vi "Getting Started with OAT (Offline, Analog Tacho) .vi"() -> ()   [LabVIEW 2017]
doc: "<B>DESCRIPTIONS</B>:\nThis VI demonstrates how to perform basic order analysis functions such as speed calculation, vibration level measurement, spectral map, order power spectrum, and order magnitude and phase. It uses simulated signals or loads previously recorded signals acquired with Log Data (Analog Tacho, DAQmx).vi for offline analysis. \n\n<B>INSTRUCTIONS</B>:\n1. Select tab page <B>Generate Signal</B> to use simulated signal or tab page <B>Load Data</B> to load logged signal.\n2. When using simulated signal, specify the <B>sampling info</B>, <B>signal rotating speed</B> and <B>order components</B> contained in the signal.\n3. When using recorded data, select the data file to load.\n4. Run the VI.\n5. On the <B>Time Waveform and Speed Profile</B> tab, select the signal of interest in <B>select channel</B> and specify the <B>Start</B> and <B>Duration</B> of the signal to calculate sound or vibration level. Run the VI again to make the changes take effect.\n6. On the <B>Colormap</B> tab, select the signal of interest in <B>select channel</B>. Use the <B>plot type</B> control to change the type of colormap. Specify the <B>time segment</B> and <B>spectra settings</B> to get a better view of the colormap. Run the VI again to make the changes take effect.\n7. On the <B>Order Power Spectrum</B> tab, specify the <B>Start</B> and <B>Duration</B> of the signal to calculate the order power spectrum. Specify the <B>window type</B>, <B>block size</B> and <B>averaging parameters</B> to improve the order power spectrum calculation and display. Run the VI again to make the changes take effect.\n<B>Note</B>: when the <B>Duration</B> of the signal is too short, there may not be an order power spectrum output. In this case, you should increase the duration or decrease the <B>block size</B> to get the order power spectrum results.\n8. On the <B>Magnitude and Phase</B> tab, select the signal of interest in <B>select channel</B> and specify the order to calculate magnitude and phase in <B>orders to compute</B>. Change the <B>magnitude view</B> and <B>view</B> to gain desired magnitude and phase display formats. Run the VI again to make the changes take effect.\n\n<B>ORDER ANALYSIS VIs USED IN THIS EXAMPLE</B>:\n1. SVL Scale Voltage to EU.vi\n2. OAT Analog Tacho Process.vi\n3. SVL RMS Level.vi\n4. SVL Peak Level.vi\n5. OAT Spectral Map.vi\n6. OAT Convert to Even Angle Signal.vi\n7. OAT Order Power Spectrum.vi\n8. OAT Order Magnitude and Phase.vi\n9. SVL Unit Conversion.vi"
uses:
  <vilib>/addons/_NISVFA/_Shared subVIs/Controls/svc_Channel Info.ctl
  <vilib>/addons/_NISVFA/_Shared subVIs/Controls/svc_Engineering Units Text Ring.ctl
  <vilib>/addons/_NISVFA/_Shared subVIs/Controls/svc_Weighting Filter Text Ring.ctl
  <vilib>/addons/_XControls/Colormap/SVX Colormap.xctl
  <vilib>/addons/_NISVFA/_Shared subVIs/Common/svc_Set SV Channel Info.vi
  <vilib>/addons/_NISVFA/_Shared subVIs/Common/svc_Set SV Channel Info (variant).vi
  <vilib>/addons/_NISVFA/_Shared subVIs/Common/SVL Set dB Reference (variant).vi
  <vilib>/addons/_NISVFA/_Shared subVIs/Common/svc_Caller VI Returned in Error Source.vi
  <vilib>/addons/_NISVFA/_Shared subVIs/Common/svc_Engineering Units to Unit Label.vi
  <vilib>/addons/_NISVFA/_Shared subVIs/Common/svc_Set dB ref if Pascal.vi
  <vilib>/addons/_NISVFA/_Shared subVIs/Common/svc_Compute Scale Factor to Convert C to EU.vi
  <vilib>/addons/_NISVFA/_Shared subVIs/Common/svc_Compute Scale Factor to Convert V to EU.vi
  <vilib>/addons/Sound and Vibration/svt_Calibration/SoundVib_Calibration.lvlib
  <vilib>/addons/Sound and Vibration/Order Analysis/Tach Process/SoundVib_TachProcess.lvlib
  <vilib>/addons/Sound and Vibration/Order Analysis/Resample Order Tracking/SoundVib_OrderTracking.lvlib
panel:
  in  "Tab Control 2":enum32{"Generate Signal", "Load Data"}(tab)
  in  "channel info":T1={"sensor sensitivity"=1000.0, "engineering units"=1, "dB reference"=1.0, "custom label"="EU", "weighting filter"=0, "pregain"=0.0} {"pregain" format="%.2f"; "weighting filter" items=["Linear", "A-weighting", "B-weighting", "C-weighting", "ITU-R 468-4", "Dolby", "CCITT", "C-message", "Wb", "Wc", "Wd", "We", "Wf", "Wh", "Wj", "Wk", "Wm", "AES17 20 kHz lowpass", "AES17 40 kHz lowpass", "AES17 20 kHz highpass", "AES17 40 kHz highpass"]; "dB reference" format="%^.1e"; "engineering units" items=["custom..."=0, "V"=1, "A"=21, "C"=30, "pC"=31, "s"=32, "-"=29, "Pa"=2, "N"=20, "g"=3, "m/s^2"=4, "m/s"=5, "m"=6, "mm/s"=12, "mm"=13, "micron/s"=14, "micron"=15, "in/s^2"=7, "in/s"=8, "in"=9, "mil/s"=10, "mil"=11, "rad/s^2"=16, "rad/s"=17, "rad"=18, "deg/s^2"=26, "deg/s"=27, "deg"=28, "RPM"=22, "cycle/s^2"=23, "Hz"=24, "cycle"=25, "strain"=19]; "sensor sensitivity" format="%#_5f"}
  in  "order components":T4(array[cluster])=[{"order"=1, "amplitude"=1.0, "phase (deg)"=0.0, "order envelop"=0}, {"order"=2, "amplitude"=0.5, "phase (deg)"=0.0, "order envelop"=2}, {"order"=3, "amplitude"=0.25, "phase (deg)"=0.0, "order envelop"=1}, {"order"=10, "amplitude"=1.0, "phase (deg)"=0.0, "order envelop"=2}] {"order envelop" items=["None", "Sine", "Triangle"]}
  in  "sampling info":T5={"sampling frequency"=10000.0, "duration [s]"=10.0} {"sampling frequency" format="%#_6p"}
  in  "signal rotating speed":u16(ring)=3 items=["3000 RPM", "1000-6000 RPM", "6000-1000 RPM", "1000-6000-1000 RPM"]
  in  "Data Path":path
  out "fs":dbl=44100.0
  out "number of samples":i32=44100
  in  "Tab Control":T6(tab)
  out "peak level [EU]":dbl format="%.2f"
  in  "Duration":dbl=1.0 format="%0.2f"
  in  "Start":dbl format="%0.2f"
  in  "select channel":u16(ring) items=["0"]
  out "RMS level [EU]":dbl format="%.2f"
  in  "max order to analyze":dbl
  out "Speed profile":cluster{"time [s]":dbl[], "speed [RPM]":dbl[]}(graph)
  out "Vibration signals":waveform(dbl)(graph)
  in  "plot type":T7(ring)
  in  "time segment [s]":T8 {"step size [s]" format="%.2f"; "end [s]" min=0.0 format="%.2f"; "start [s]" min=0.0 format="%.2f"}
  in  "select channel":u16(ring) items=["0"]
  in  "spectral settings":T9={"window type"=62, "freq/order bins"=2048} {"freq/order bins" min=2; "window type" items=["None"=0, "Hanning"=1, "Hamming"=2, "Blackman-Harris"=3, "Exact Blackman"=4, "Blackman"=5, "Flat Top"=6, "4 Term B-Harris"=7, "7 Term B-Harris"=8, "Low Sidelobe"=9, "Gaussian"=62]}
  in  "dB on (T)":bool=TRUE
  out "Colormap":T10(xcontrol)
  in  "Duration [s]":dbl=10.0 format="%0.2f"
  in  "Start [s]":dbl format="%0.2f"
  in  "averaging parameters":T11={"averaging mode"=enum."RMS averaging", "weighting mode"=enum."Exponential", "number of averages"=10, "linear mode"=enum."One shot"} {"number of averages" min=1 step=1}
  in  "block size":i32=1024 min=2
  in  "window type":u32(ring)=1 items=["None"=0, "Hanning"=1, "Hamming"=2, "Blackman-Harris"=3, "Exact Blackman"=4, "Blackman"=5, "Flat Top"=6, "4 Term B-Harris"=7, "7 Term B-Harris"=8, "Low Sidelobe"=9, "Gaussian"=62]
  in  "dB On":bool=TRUE
  out "Order Power Spectrum":T12(graph) caption="Order power spectrum"
  in  "view":T13={"dB on? (F)"=FALSE, "unwrap phase? (T)"=TRUE, "unit in degree? (T)"=TRUE}
  in  "magnitude view":enum16{"no change", "rms", "peak", "peak-peak"}(ring)
  in  "select channel":u16(ring) items=["0"]
  in  "X axis selection":u16(ring) items=["Time", "Revolution", "RPM"]
  in  "bandwidth [order]":dbl format="%.2f"
  in  "orders to compute":dbl[](array[numeric])=[1.0] format="%.2f"
  out "Phase":cluster{"time/rev/rpm":dbl[], "phase":dbl[]}[](graph)
  out "Magnitude":T14(graph)
  # "Select Help»Show Context Help and move the cursor over the VI icon for more information."
  # "Sound or Vibration Level Measurement"
  # "select data block"
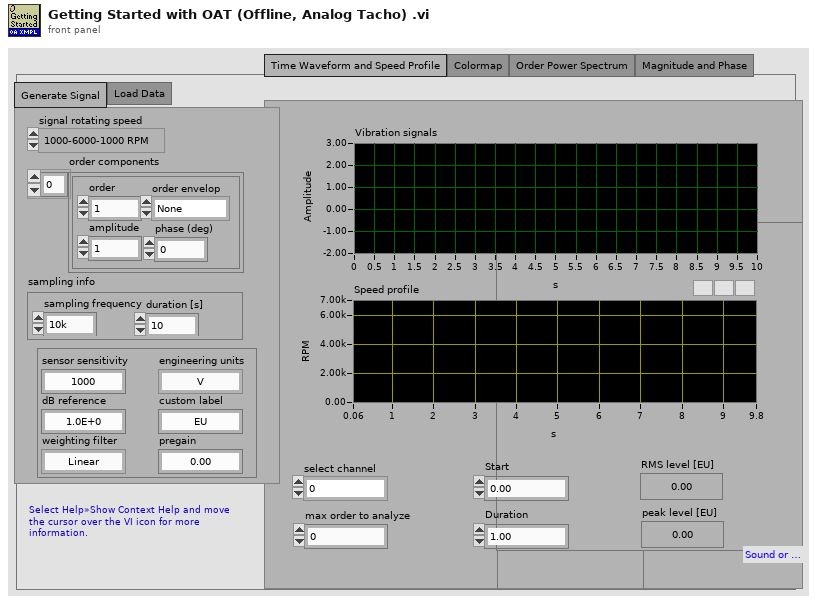
[diagram p1: front panel]
types:
  T1 = typedef "svc_Channel Info.ctl" = cluster{"sensor sensitivity":dbl, "engineering units":T2, "dB reference":dbl, "custom label":string, "weighting filter":T3, "pregain":dbl}
  T2 = typedef "svc_Engineering Units Text Ring.ctl" = u16
  T3 = typedef "svc_Weighting Filter Text Ring.ctl" = u16
  T4 = cluster{"order":i32, "amplitude":dbl, "phase (deg)":dbl, "order envelop":u16}[]
  T5 = cluster{"sampling frequency":dbl, "duration [s]":dbl}
  T6 = enum32{"Time Waveform and Speed Profile", "Colormap", "Order Power Spectrum", "Magnitude and Phase"}
  T7 = enum16{"Frequency-Time", "Time-Frequency", "Order-Time", "Time-Order", "Frequency-RPM", "RPM-Frequency", "Order-RPM", "RPM-Order"}
  T8 = cluster{"start [s]":dbl, "end [s]":dbl, "step size [s]":dbl}
  T9 = cluster{"window type":u32, "freq/order bins":i32}
  T10 = cluster{"spectral map":dbl[][], "X scale":cluster{"offset":dbl, "multiplier":dbl}, "Y scale":cluster{"offset":dbl, "multiplier":dbl}, "attribute":variant}
  T11 = cluster{"averaging mode":enum16{"No averaging", "Vector averaging", "RMS averaging", "Peak hold"}, "weighting mode":enum16{"Linear", "Exponential"}, "number of averages":u32, "linear mode":enum16{"One shot", "Auto restart"}}
  T12 = cluster{"order 0":dbl, "delta order":dbl, "magnitude":dbl[]}[]
  T13 = cluster{"dB on? (F)":bool, "unwrap phase? (T)":bool, "unit in degree? (T)":bool}
  T14 = cluster{"time/rev/rpm":dbl[], "magnitude":dbl[]}[]
  T15 = cluster{"pulse / rev":i32, "threshold (auto)":dbl, "slope (Rising)":u16}
  T16 = typedef "SoundVib_TachProcess.lvlib/speed profile.ctl" = cluster{"time [s]":dbl[], "speed [RPM]":dbl[]}
  T17 = cluster{"value":dbl[][], "x scale":cluster{"offset":dbl, "multiplier":dbl}, "y scale":cluster{"offset":dbl, "multiplier":dbl}, "attribute":variant}
  T18 = cluster{"x-axis unit label":string, "y-axis unit label":string, "z-axis unit label":string}
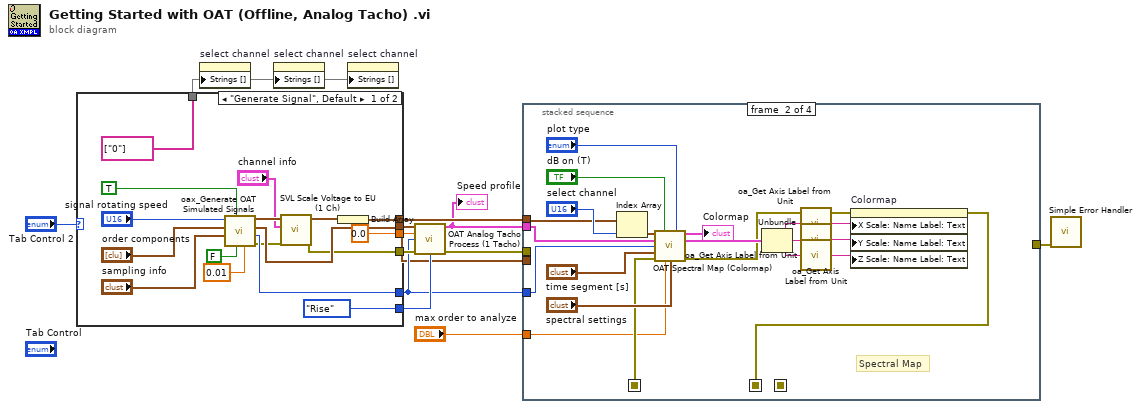
[diagram p0: block diagram]
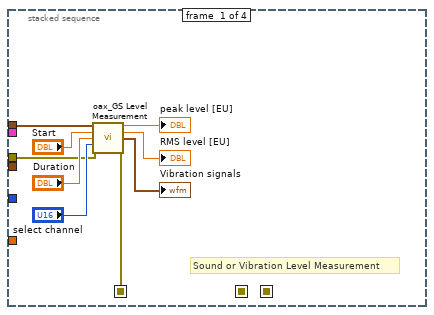
[diagram p2: hidden frame]
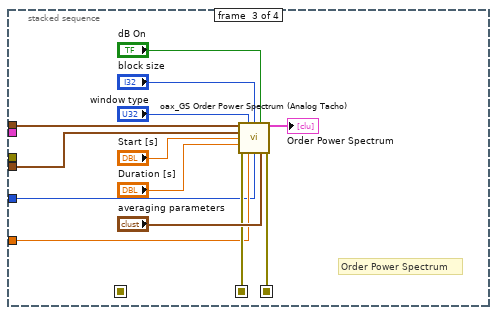
[diagram p3: hidden frame]
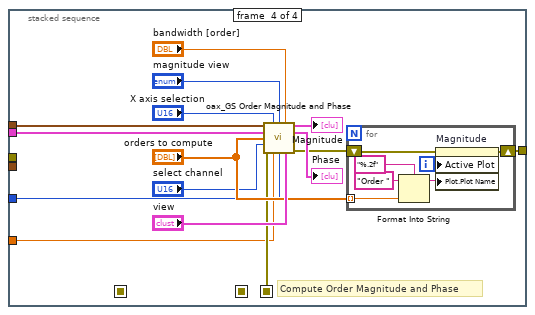
[diagram p4: hidden frame]
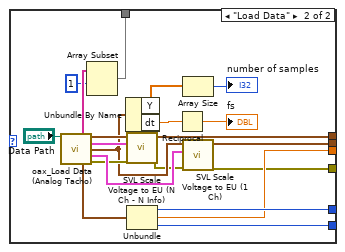
[diagram p5: hidden frame]
diagram:
  n1 = case shown="\"Generate Signal\", Default" "Tab Control 2" {
    tunnel: [w23 w44] -> w7
    tunnel: [w20 w38] -> w2
    tunnel: [w19 w42] -> w4
    tunnel: [enum16{"Rise", "Fall"}."Rise" ("slope (Rise)") w41] -> w11
    tunnel: [0.0 ("threshold (auto)") w40] -> w10
    tunnel: [string[] ["0"] w34] -> w9
    tunnel: [w13 w30] -> w8
    frame "Generate Signal", Default {
      n2 = call <vilib>:"oax_Generate OAT Simulated Signals.vi"("noise level"=0.01, "add noise?"=FALSE, "reset?"=TRUE, "sampling info"="sampling info", "ordercomponents"="order components", "signal rotating speed"="signal rotating speed") -> ("error out"=w18:errorcluster, "pulse/revolution"=w19:i32, "Tach Signal"=w20:waveform(dbl), "Vibration Signal"=w22:waveform(dbl))  [unwired: 2 in]
      n3 = call <vilib>:"SVL Scale Voltage to EU (1 Ch).vi"("error in (no error)"=w18, "channel info"="channel info", "signal [V]"=w22) -> ("error out"=w13:errorcluster, "scaled signal [EU]"=w21:waveform(dbl))  [unwired: 6 in, 1 out]
      n4 = Build Array(w21) -> (w23:waveform(dbl)[])
    }
    frame "Load Data" {
      n5 = call <vilib>:"oax_Load Data (Analog Tacho).vi"("Data Path In"="Data Path") -> ("channel name"=w36:string[], "vibration data"=w45:waveform(dbl)[], "vibration channel info"=w33:T1[], "analog tacho signal"=w32:waveform(dbl), "tacho channel info"=w39:T1, "tacho info"=w43:T15, "error out"=w37:errorcluster)  [unwired: 8 in]
      n6 = Array Subset(array=w36, index=1) -> (w34:string[])  [unwired: 1 in]
      n7 = Unbundle By Name(w32) -> ("Y"=w47:dbl[], "dt"=w49:dbl)
      n8 = call <vilib>:"SVL Scale Voltage to EU (N Ch - N Info).vi"("error in (no error)"=w37, "channel info"=w33, "signals [V]"=w45) -> ("error out"=w31:errorcluster, "scaled signals [EU]"=w44:waveform(dbl)[])  [unwired: 6 in, 1 out]
      n9 = Unbundle(w43) -> ("pulse / rev"=w42:i32, "threshold (auto)"=w40:dbl, "slope (Rising)"=w41:u16)
      n10 = Reciprocal(x=w49) -> (1/x=→"fs":dbl)
      n11 = Array Size(array=w47) -> (size(s)=→"number of samples":i32)
      n12 = call <vilib>:"SVL Scale Voltage to EU (1 Ch).vi"("error in (no error)"=w31, "channel info"=w39, "signal [V]"=w32) -> ("error out"=w30:errorcluster, "scaled signal [EU]"=w38:waveform(dbl))  [unwired: 6 in, 1 out]
    }
  }
  n13 = property on="select channel" class="Ring (strict)"("Strings []"=w9) -> ()  [unwired: 2 in, 2 out]
  n14 = property on="select channel" class="Ring (strict)"("Strings []"=w9) -> ()  [unwired: 2 in, 2 out]
  n15 = property on="select channel" class="Ring (strict)"("Strings []"=w9) -> ()  [unwired: 2 in, 2 out]
  n16 = call <vilib>:"OAT Analog Tacho Process (1 Tacho).vi"("analog tacho signal"=w2, "threshold (auto)"=w10, "pulse/revolution (1)"=w4, "error in (no error)"=w8, "slope (Rising)"=w11) -> ("speed profile"=w5:T16, "error out"=w6:errorcluster)  [unwired: 6 in, 3 out]
  "Speed profile" <- w5
  n17 = stacked-sequence {
    seq-local: [w51 _ _ _] -> [_ w74 _ _]
    seq-local: [_ w67 _ _] -> [_ _ w85 _]
    seq-local: [_ _ w81 _] -> [_ _ _ w98]
    tunnel: w7 -> [w53 w75 w86 w100]
    tunnel: w6 -> [w52 _ _ _]
    tunnel: w5 -> [_ w73 _ w99]
    tunnel: w4 -> [_ w72 w82 w96]
    tunnel: "max order to analyze" -> [_ w71 w83 w97]
    tunnel: w2 -> [_ _ w84 _]
    tunnel: [_ _ _ w94] -> w1
    frame #0 {
      # "Sound or Vibration Level Measurement"
      n18 = call <vilib>:"oax_GS Level Measurement.vi"("scaled signals [EU]"=w53, "Start"="Start", "Duration"="Duration", "select channel"="select channel", "error in (no error)"=w52) -> ("Peak level [EU]"=→"peak level [EU]":dbl, "RMS level [EU]"=→"RMS level [EU]":dbl, "vibration signals"=→"Vibration signals":waveform(dbl), "error out"=w51:errorcluster)  [unwired: 7 in]
    }
    frame #1 {
      # "Spectral Map"
      n19 = Index Array(array=w75, index="select channel") -> (element=w77:waveform(dbl))
      n20 = call <vilib>:"OAT Spectral Map (Colormap).vi"("scaled signal [EU]"=w77, "dB on? (T)"="dB on (T)", "plot type"="plot type", "speed profile"=w73, "pulse/revolution (1)"=w72, "time/speed segment [s or RPM]"="time segment [s]", "error in (no error)"=w74, "max order (auto)"=w71, "windows info"="spectral settings") -> ("colormap"=→"Colormap":T17, "colormap unit labels"=w69:T18, "error out"=w68:errorcluster)  [unwired: 2 in, 2 out]
      n21 = Unbundle(w69) -> ("x-axis unit label"=w63:string, "y-axis unit label"=w65:string, "z-axis unit label"=w61:string)
      n22 = call <vilib>:"oa_Get Axis Label from Unit.vi"("Unit"=w63) -> ("Label"=w62:string)  [unwired: 4 in]
      n23 = call <vilib>:"oa_Get Axis Label from Unit.vi"("Unit"=w65) -> ("Label"=w64:string)  [unwired: 4 in]
      n24 = call <vilib>:"oa_Get Axis Label from Unit.vi"("Unit"=w61) -> ("Label"=w60:string)  [unwired: 4 in]
      n25 = property on="Colormap" class="Colormap (strict)"(error in=w68, "X Scale: Name Label: Text"=w62, "Y Scale: Name Label: Text"=w64, "Z Scale: Name Label: Text"=w60) -> (error out=w67:errorcluster)  [unwired: 1 in, 1 out]
    }
    frame #2 {
      # "Order Power Spectrum"
      n26 = call <vilib>:"oax_GS Order Power Spectrum (Analog Tacho).vi"("scaled signals [EU]"=w86, "window type"="window type", "block size"="block size", "dB On"="dB On", "Waveform"=w84, "Start"="Start [s]", "Duration"="Duration [s]", "error in (no error)"=w85, "max order to analyze"=w83, "pulse/rev"=w82, "averaging parameters"="averaging parameters") -> ("Order Power Spectrum"=→"Order Power Spectrum":T12, "error out"=w81:errorcluster)  [unwired: 3 in]
    }
    frame #3 {
      # "Compute Order Magnitude and Phase"
      n27 = call <vilib>:"oax_GS Order Magnitude and Phase.vi"("scaled signals [EU]"=w100, "X axis selection"="X axis selection", "magnitude view"="magnitude view", "bandwidth [order]"="bandwidth [order]", "speed profile"=w99, "orders to track"="orders to compute", "select channel"="select channel", "error in (no error)"=w98, "max order to analyze"=w97, "pulse/rev"=w96, "view"="view") -> ("magnitude"=→"Magnitude":T14, "phase"=→"Phase":cluster{"time/rev/rpm":dbl[], "phase":dbl[]}[], "error out"=w95:errorcluster)  [unwired: 1 in, 1 out]
      n28 = for {
        tunnel: "orders to compute" -> [w115] mode=indexing
        shift-right: [w109] -> w94
        shift-left: w95 -> [w110]
        i -> [w111]
        n29 = Format Into String(format string="%.2f" ("Format String"), initial string="Order " ("Input String"), w115) -> (resulting string=w112:string)  [unwired: 1 in, 1 out]
        n30 = property on="Magnitude" class="XYGraph (strict)"(error in=w110, "Active Plot"=w111, "Plot.Plot Name"=w112) -> (error out=w109:errorcluster)  [unwired: 1 in, 1 out]
      }
    }
  }
  n31 = call <vilib>:"Simple Error Handler.vi"("error in (no error)"=w1) -> ()  [unwired: 4 in, 5 out]
